vi "PatternMatching.vi"(0 "Image In":T1, 1 "Image Dst":T1, 2 "ROI Descriptor (Pattern Matching 1)":T2={"Global Rectangle"=[20, 20, 620, 460], "Contours"=[{"ID"=enum."External", "Type"=12, "Coordinates"=[20, 20, 620, 460, 0]}]} {"Contours"."Type" items=["No Selection", "Point", "Line", "Rectangle", "Oval", "Polygon", "Freehand Region", "Annulus", "Unused2", "Unused3", "Broken Line", "Freehand Line", "Rotated Rectangle"]}, 3 "Match Mode (Pattern Matching 1)":u16(ring)=1 items=["Shift Invariant", "Rotation Invariant"], 4 "Number of Matches Requested (Pattern Matching 1)":i32=1, 5 "Minimum Match Score (Pattern Matching 1)":sgl=300.0, 6 "Subpixel Accuracy (Pattern Matching 1)":bool, 7 "error in":errorcluster, 8 "Rotation Angle Ranges (degrees) (Pattern Matching 1)":cluster{sgl, sgl}[](array[cluster])=[{-20.0, 20.0}], 9 "Match Offset (Pattern Matching 1)":cluster{"X":sgl, "Y":sgl}, 10 "Marker Image":T1) -> (20 "Image Out":T1(plugin-control), 21 "Matches (Pattern Matching 1)":T3(array[cluster]) {"Bounding Box"."y" format="%.2f"; "Bounding Box"."x" format="%.2f"; "Position"."y" format="%.2f"; "Position"."x" format="%.2f"; "Score" format="%.2f"; "Scale" format="%.2f"; "Angle" format="%.2f"}, 22 "Calibrated Matches (Pattern Matching 1)":T3(array[cluster]) {"Bounding Box"."y" format="%.2f"; "Bounding Box"."x" format="%.2f"; "Position"."y" format="%.2f"; "Position"."x" format="%.2f"; "Score" format="%.2f"; "Scale" format="%.2f"; "Angle" format="%.2f"}, 23 "Number of Matches (Pattern Matching 1)":i32, 27 "error out":errorcluster)   [LabVIEW 2013]
doc: "Creates, edits, and runs vision algorithms using NI Vision Assistant.\n\nWhen you place this Express VI on the block diagram, NI Vision Assistant launches. Create an algorithm using the Vision Assistant processing functions. After you create an algorithm, you can select the controls and indicators that you want to be able to programmatically set in LabVIEW. Double-click the Vision Assistant Express VI to edit the algorithm."
uses:
  <vilib>/vision/Image Controls.llb/IMAQ Image.ctl
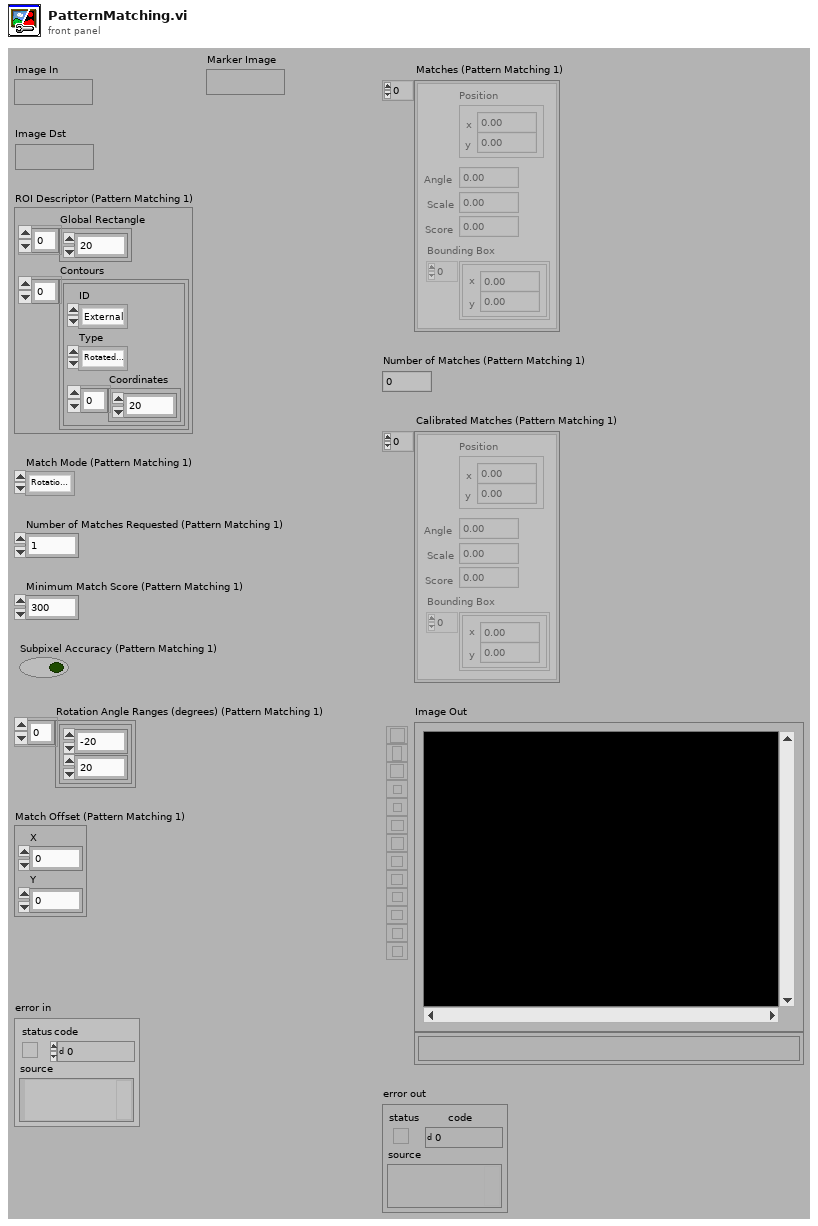
[diagram p1: front panel]
types:
  T1 = typedef "IMAQ Image.ctl" = refnum<image>
  T2 = cluster{"Global Rectangle":i32[], "Contours":cluster{"ID":enum32{"External", "Internal"}, "Type":u32, "Coordinates":i32[]}[]}
  T3 = cluster{"Position":cluster{"x":sgl, "y":sgl}, "Angle":sgl, "Scale":sgl, "Score":sgl, "Bounding Box":cluster{"x":sgl, "y":sgl}[]}[]
  T4 = typedef "Image Type" = u32
  T5 = cluster{"Match Mode (Pattern Matching 1)":u16, "Subpixel Accuracy (Pattern Matching 1)":bool, "Rotation Angle Ranges (degrees) (Pattern Matching 1)":cluster{sgl, sgl}[]}
  T6 = cluster{"ROI Descriptor (Pattern Matching 1)":cluster{"Global Rectangle":i32[], "Contours":cluster{"ID":enum32{"External", "Internal"}, "Type":u32, "Coordinates":i32[]}[]}, "Number of Matches Requested (Pattern Matching 1)":i32, "Minimum Match Score (Pattern Matching 1)":sgl}
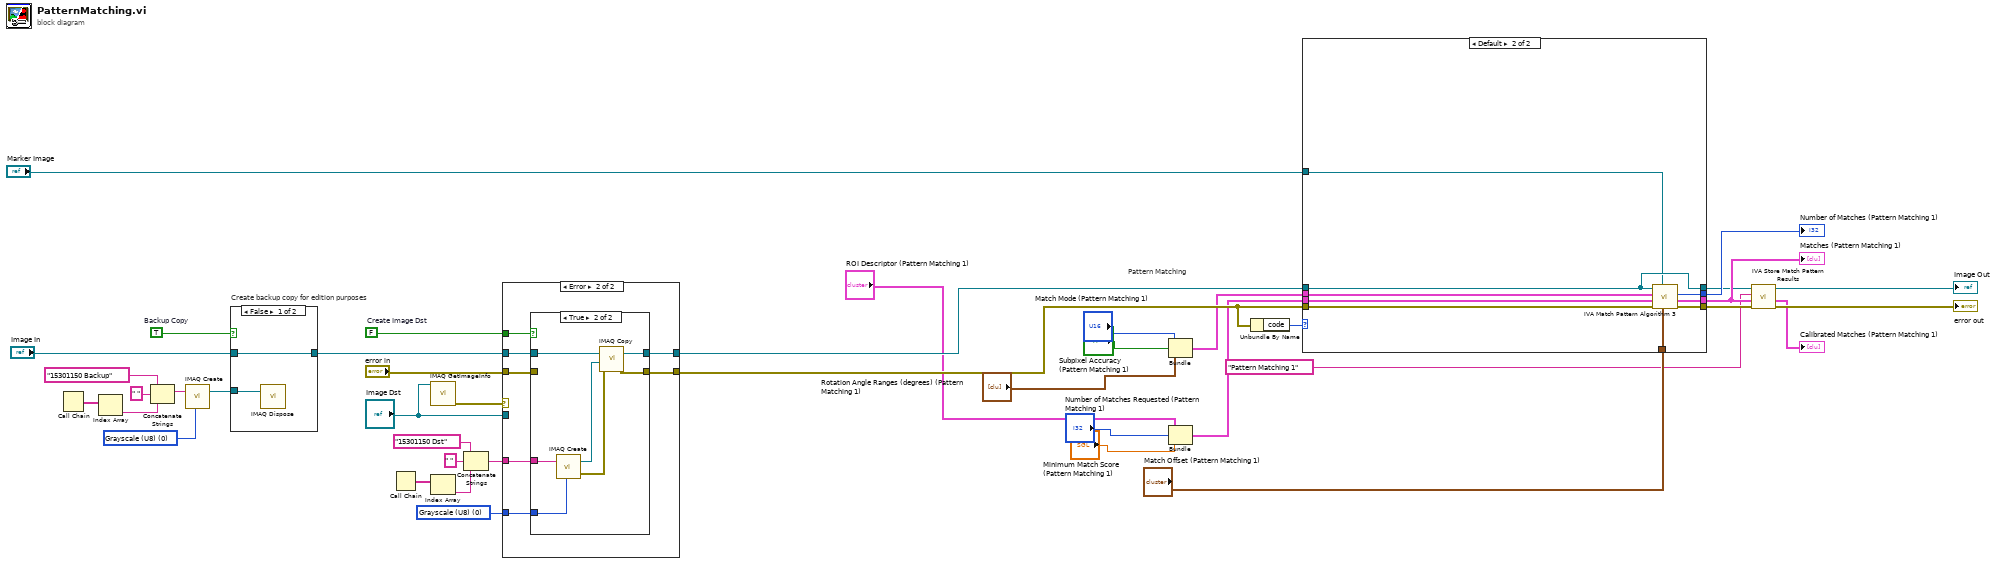
[diagram p0: block diagram]
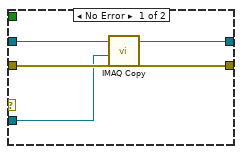
[diagram p3: hidden frame]
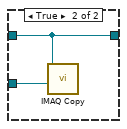
[diagram p5: hidden frame]
diagram:
  w21 = T4 0 items=["Grayscale (U8)", "Grayscale (I16)", "Grayscale (SGL)", "Complex (CSG)", "RGB (U32)", "HSL (U32)", "RGB (U64)", "Grayscale (U16)"] ("Image Dst Type")
  w22 = T4 0 items=["Grayscale (U8)", "Grayscale (I16)", "Grayscale (SGL)", "Complex (CSG)", "RGB (U32)", "HSL (U32)", "RGB (U64)", "Grayscale (U16)"] ("Image Type")
  w41 = TRUE  # Backup Copy
  w34 = FALSE  # Create Image Dst
  # "Pattern Matching"
  n1 = Call Chain() -> (call chain=w28:string[])
  n2 = Index Array(array=w28) -> (element=w27:string)  [unwired: 1 in]
  n3 = Concatenate Strings("15301150 Backup" ("Backup Image Name"), " ", w27) -> (w24:string)
  n4 = call "IMAQ Create"("Image Name"=w24, "Image Type"=w22) -> ("New Image"=w23:T1)  [unwired: 2 in, 2 out]
  n5 = case "Create backup copy for edition purposes" shown="False" w41 {
    tunnel: [w43 w45] -> w37
    tunnel: "Image In" -> [w43 w45]
    tunnel: w23 -> [w42 w44]
    frame False {
      n6 = call "IMAQ Dispose"("Image"=w42) -> ()  [unwired: 2 in, 4 out]
    }
    frame True {
      n7 = call "IMAQ Copy"("Image Dst"=w44, "Image Src"=w45) -> ()  [unwired: 1 in, 5 out]
    }
  }
  n8 = Call Chain() -> (call chain=w33:string[])
  n9 = call "IMAQ GetImageInfo"("Image"="Image Dst") -> ("error out"=w39:errorcluster)  [unwired: 1 in, 9 out]
  n10 = Index Array(array=w33) -> (element=w31:string)  [unwired: 1 in]
  n11 = Concatenate Strings("15301150 Dst" ("Image Dst Name"), " ", w31) -> (w29:string)
  n12 = case shown="Error" w39 {
    tunnel: [w50 w54] -> w11
    tunnel: [w49 w53] -> w35
    tunnel: w37 -> [w48 w55]
    tunnel: "error in" -> [w47 w51]
    tunnel: "Image Dst" -> [w46 _]
    tunnel: w29 -> [_ w57]
    tunnel: w21 -> [_ w56]
    tunnel: w34 -> [_ w52]
    frame No Error {
      n13 = call "IMAQ Copy"("error in (no error)"=w47, "Image Dst"=w46, "Image Src"=w48) -> ("error out"=w49:errorcluster, "Image Dst Out"=w50:T1)  [unwired: 3 out]
    }
    frame Error {
      n14 = case shown="True" w52 {
        tunnel: w57 -> [_ w66]
        tunnel: w56 -> [_ w65]
        tunnel: w55 -> [w59 w63]
        tunnel: [w59 w62] -> w54
        tunnel: [w58 w61] -> w53
        tunnel: w51 -> [w58 _]
        frame False {
        }
        frame True {
          n15 = call "IMAQ Create"("Image Name"=w66, "Image Type"=w65) -> ("New Image"=w64:T1, "error out"=w60:errorcluster)  [unwired: 2 in, 1 out]
          n16 = call "IMAQ Copy"("error in (no error)"=w60, "Image Dst"=w64, "Image Src"=w63) -> ("error out"=w61:errorcluster, "Image Dst Out"=w62:T1)  [unwired: 3 out]
        }
      }
    }
  }
  n17 = Bundle("Match Mode (Pattern Matching 1)"="Match Mode (Pattern Matching 1)", "Subpixel Accuracy (Pattern Matching 1)"="Subpixel Accuracy (Pattern Matching 1)", "Rotation Angle Ranges (degrees) (Pattern Matching 1)"="Rotation Angle Ranges (degrees) (Pattern Matching 1)") -> (w16:T5)  [unwired: 1 out]
  n18 = Bundle("ROI Descriptor (Pattern Matching 1)"="ROI Descriptor (Pattern Matching 1)", "Number of Matches Requested (Pattern Matching 1)"="Number of Matches Requested (Pattern Matching 1)", "Minimum Match Score (Pattern Matching 1)"="Minimum Match Score (Pattern Matching 1)") -> (w13:T6)  [unwired: 1 out]
  n19 = Unbundle By Name(w35) -> ("code"=w5:i32)
  n20 = case shown="Default" w5 {
    tunnel: w35 -> [_ w69]
    tunnel: [_ w76] -> w20
    tunnel: w16 -> [_ w75]
    tunnel: w13 -> [_ w74]
    tunnel: "Match Offset (Pattern Matching 1)" -> [_ w73]
    tunnel: w11 -> [w67 w70]
    tunnel: [_ w72] -> w10
    tunnel: [_ w71] -> w7
    tunnel: [w67 w70] -> w6
    tunnel: "Marker Image" -> [_ w68]
    frame -1074396199, -1074396198 {
      # "Discard\nCoordinate\nSystem Error"
    }
    frame Default {
      n21 = call <vilib>:"IVA Match Pattern Algorithm 3.vi"("Match Offset"=w73, "Image Template"=w68, "error in (no error)"=w69, "Match Parameters"=w74, "Setup Match Parameters"=w75, "Image"=w70) -> ("error out"=w72:errorcluster, "Number of Matches"=w76:i32, "Matches"=w71:T3)  [unwired: 3 out]
    }
  }
  "Matches (Pattern Matching 1)" <- w7
  "Number of Matches (Pattern Matching 1)" <- w20
  n22 = call <vilib>:"IVA Store Match Pattern Results.vi"("error in (no error)"=w10, "Matches"=w7, "Step Name"="Pattern Matching 1", "Image in"=w6) -> ("error out"=→"error out":errorcluster, "Calibrated Matches"=→"Calibrated Matches (Pattern Matching 1)":T3, "Image dup"=→"Image Out":T1)  [unwired: 5 out]
